vi "Init.vi"(8 "error in (no error)":errorcluster, 9 "Constant Action Data":string, 10 "HAL GOOP4.lvlib:Instrument Base":refnum<class "Instr Base.lvclass">, 11 "Virt Voltage Reader in":refnum<class "Virt Voltage Reader.lvclass">) -> (0 "error out":errorcluster, 3 "Virt Voltage Reader out":refnum<class "Virt Voltage Reader.lvclass">)   [LabVIEW 2023, in "Virt Scopes.lvlib" / "Virt Voltage Reader.lvclass"]
uses:
  Virt Voltage Reader.lvclass
  D:/git/HAL/HAL GOOP4/Virt Instrument Base/Virt Instr Base.lvclass
  Instrument Base/Instr Base.lvclass
  Virt Instrument Base/Virt Instr Base.lvclass/Virt Instr Base.ctl
  Virt Voltage Reader.lvclass/Virt Voltage Reader.ctl
  Virt Instrument Base/Virt Instr Base.lvclass
  D:/git/HAL/HAL GOOP4/Scope/Virtual Scopes/Virt Voltage Reader/Virtual Voltage Reader/Virt Voltage Reader.lvclass
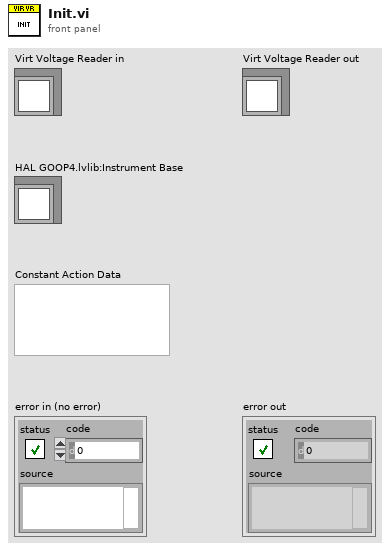
[diagram p1: front panel]
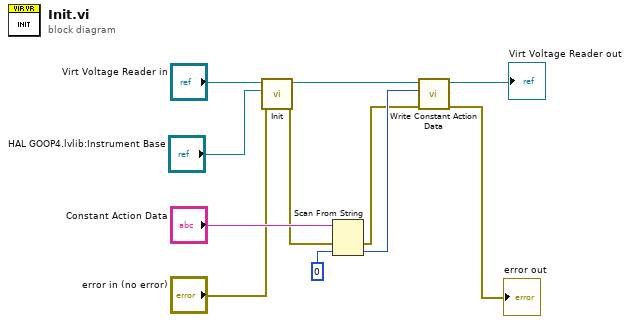
[diagram p0: block diagram]
diagram:
  n1 = call-parent "Init.vi"("error in (no error)"="error in (no error)", "HAL GOOP4.lvlib:Instrument Base"="HAL GOOP4.lvlib:Instrument Base", "Virt Instrument Base in"="Virt Voltage Reader in") -> ("error out"=w4:errorcluster, "Virt Instrument Base out"=w2:refnum<class "Virt Voltage Reader.lvclass">)  [unwired: 7 in]
  n2 = Scan From String(input string="Constant Action Data", error in=w4, default 1=u8 0) -> (error out=w6:errorcluster, output 1=w8:u8)  [unwired: 2 in, 2 out]
  n3 = call "Write Constant Action Data.vi"("error in (no error)"=w6, "Constant Action Data"=w8, "Virt Instrument Base in"=w2) -> ("error out"=→"error out":errorcluster, "Virt Instrument Base out"=→"Virt Voltage Reader out":refnum<class "Virt Voltage Reader.lvclass">)  [unwired: 7 in]
